vi "Init3478.vi"(2 "error in (no error)":errorcluster, 3 "VISA session 2":refnum<visa-resource-name>) -> (0 "error out":errorcluster, 1 "VISA session":refnum<visa-resource-name>)   [LabVIEW 2012]
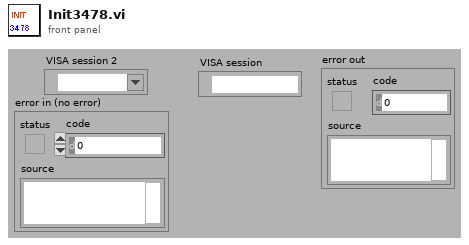
[diagram p1: front panel]
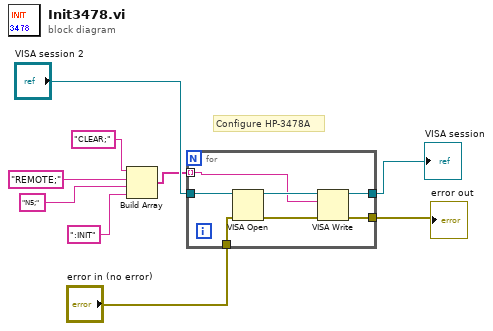
[diagram p0: block diagram]
diagram:
  # "Configure HP-3478A"
  n1 = Build Array("CLEAR;", "REMOTE;", "N5;", ":INIT" ("element")) -> (w5:string[])
  n2 = for {
    tunnel: w5 -> [w14] mode=indexing
    tunnel: "VISA session 2" -> [w16]
    tunnel: [w12] -> w8
    tunnel: [w11] -> w9
    tunnel: "error in (no error)" -> [w10]
    n3 = VISA Open(error in (no error)=w10, VISA resource name=w16) -> (VISA resource name=w15:refnum<visa-resource-name>, error out=w13:errorcluster)  [unwired: 3 in]
    n4 = VISA Write(VISA resource name=w15, write buffer=w14, error in (no error)=w13) -> (VISA resource name out=w12:refnum<visa-resource-name>, error out=w11:errorcluster)  [unwired: 1 out]
  }
  "error out" <- w9
  "VISA session" <- w8
